vi "UDT_admittanceLibrary_tf FGV.vi"() -> (3 "Unit Test Framework Results":T1)   [LabVIEW 2017]
doc: "Use this template to create a user-defined test VI. Define your test requirements and wire the results to the <b>Result (Test)</b> control. Do not modify the <b>Unit Test Framework Results</b> indicator."
uses:
  <vilib>/utf/common/utf_test_result_troll.ctl
  <vilib>/utf/common/utf_test_result.ctl
  <vilib>/utf/common/utf_test_result_failure.ctl
  <vilib>/utf/common/utf_test_comparison_operators.ctl
  <vilib>/utf/common/utf_vi_tag.ctl
  RT/Admittance Controller/Controls/tf control.ctl
  <vilib>/Control Software Solutions Ltd/UTF Helper/SubVIs/UTF Double Not Equals.vi
  <vilib>/Control Software Solutions Ltd/UTF Helper/SubVIs/UTF Double Equals.vi
  <vilib>/Control Software Solutions Ltd/UTF Helper/Unit Test Helper.lvlib
  RT/Admittance Controller/admittanceControllerLibrary.lvlib
  <vilib>/utf/NI_UnitTestFramework.lvlib
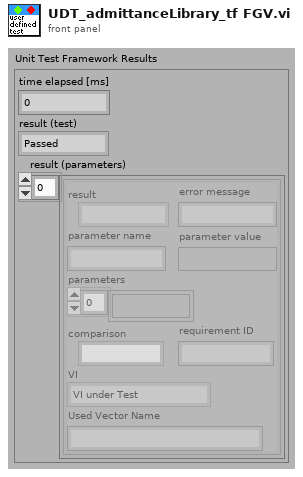
[diagram p1: front panel]
types:
  T1 = typedef "NI_UnitTestFramework.lvlib/utf_test_result_troll.ctl" = cluster{"time elapsed [ms]":u32, "result (test)":T2, "result (parameters)":T3[]}
  T2 = typedef "NI_UnitTestFramework.lvlib/utf_test_result.ctl" = enum16{"Passed", "Failed", "Error", "Skipped", "Not Processed"}
  T3 = typedef "NI_UnitTestFramework.lvlib/utf_test_result_failure.ctl" = cluster{"result":T2, "error message":string, "parameter name":string, "parameter value":variant, "parameters":variant[], "comparison":T4, "requirement ID":string, "VI":T5, "Used Vector Name":string}
  T4 = typedef "NI_UnitTestFramework.lvlib/utf_test_comparison_operators.ctl" = enum16{"=", "!=", ">", ">=", "<", "<=", "range", "symmetric tolerance", "asymmetric tolerance", "string contains", "string not contain", "array size", "string length", "array range", "by element", "array range (limit array)", "user-defined", "array contains", "array not contain", "vector length", "= (elm)", "!= (elm)", "= (case insensitive)", "!= (case insensitive)"}
  T5 = typedef "NI_UnitTestFramework.lvlib/utf_vi_tag.ctl" = enum16{"Setup VI", "VI under Test", "Teardown VI"}
  T6 = typedef "admittanceControllerLibrary.lvlib/tf control.ctl" = enum16{"get tf", "set tf"}
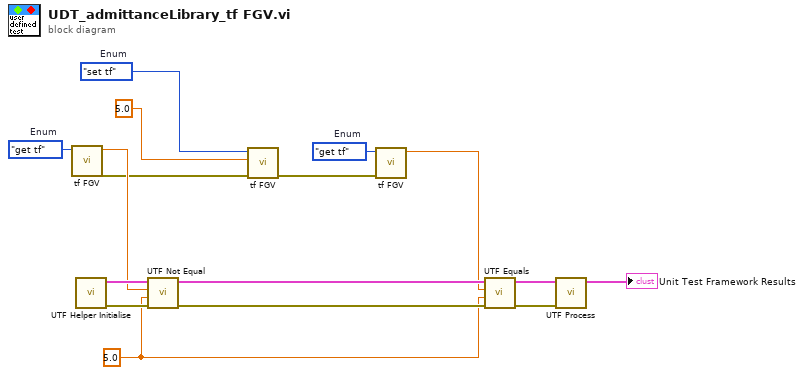
[diagram p0: block diagram]
diagram:
  w3 = tf_control."get tf"  # Enum
  w6 = tf_control."set tf"  # Enum
  w9 = tf_control."get tf"  # Enum
  w12 = 5.0 ("X0")
  n1 = call "tf FGV.vi"("Enum"=w9) -> ("error out"=w7:errorcluster, "tf"=w8:dbl)  [unwired: 9 in]
  n2 = call <vilib>:"UTF Helper Initialise.vi"() -> ("error out"=w15:errorcluster, "results array"=w16:T3[])  [unwired: 10 in]
  n3 = call-poly <vilib>:"UTF Not Equal.vi"("error in (no error)"=w15, "Test Value"=w12, "Input"=w8, "Input Results"=w16) -> ("error out"=w14:errorcluster, "Output Results"=w13:T3[])  [unwired: 6 in]
  n4 = call "tf FGV.vi"("error in (no error)"=w7, "set tf"=5.0 ("X0"), "Enum"=w6) -> ("error out"=w4:errorcluster)  [unwired: 7 in, 1 out]
  n5 = call "tf FGV.vi"("error in (no error)"=w4, "Enum"=w3) -> ("tf"=w2:dbl)  [unwired: 8 in, 1 out]
  n6 = call-poly <vilib>:"UTF Equals.vi"("error in (no error)"=w14, "Test Value"=w12, "Input"=w2, "Input Results"=w13) -> ("error out"=w10:errorcluster, "Output Results"=w11:T3[])  [unwired: 6 in]
  n7 = call <vilib>:"UTF Process.vi"("error in (no error)"=w10, "results array"=w11) -> ("Unit Test Framework Results"=→"Unit Test Framework Results":T1)  [unwired: 9 in]
